vi "Write zmax.vi"(8 "error in (no error)":errorcluster, 10 "zmax":i64, 11 "Cube in":refnum<class "Cube.lvclass">) -> (0 "error out":errorcluster, 3 "Cube out":refnum<class "Cube.lvclass">)   [LabVIEW 2019, in "22.lvlib" / "Cube.lvclass"]
uses:
  Cube.lvclass
  Cube.lvclass/Cube.ctl
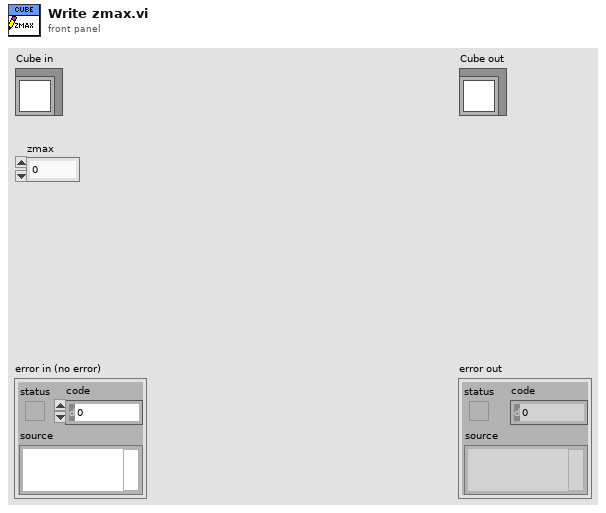
[diagram p1: front panel]
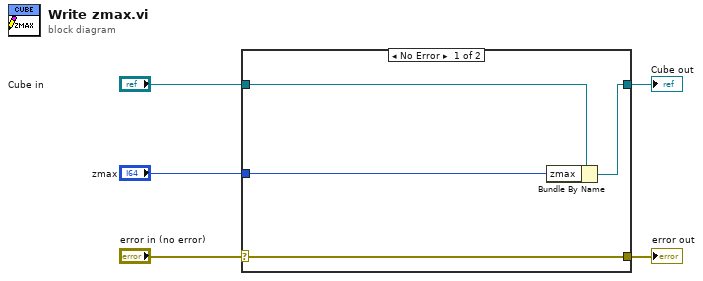
[diagram p0: block diagram]
diagram:
  n1 = case shown="No Error" "error in (no error)" {
    selector: "error in (no error)" -> [w9 w10]
    tunnel: [w9 w10] -> w4
    tunnel: [w7 w11] -> w2
    tunnel: "Cube in" -> [w8 w11]
    tunnel: "zmax" -> [w6 _]
    frame No Error {
      n2 = Bundle By Name(cluster=w8, "zmax"=w6) -> (w7:refnum<class "Cube.lvclass">)
    }
    frame Error {
    }
  }
  "error out" <- w4
  "Cube out" <- w2
